vi "T_At_Wire_Err.vi"(8 "InitClock(ms)":u32, 11 "error in (no error)":errorcluster caption="entrée d'erreur") -> (0 "Clock(ms)":u32, 3 "error out":errorcluster caption="sortie d'erreur", 4 "Delta(ms)":u32)   [LabVIEW 2019]
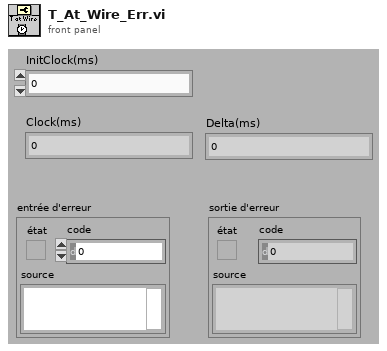
[diagram p1: front panel]
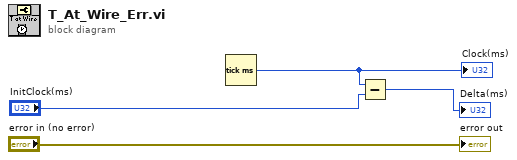
[diagram p0: block diagram]
diagram:
  n1 = Tick Count (ms)() -> (millisecond timer value=w2:u32)
  "Clock(ms)" <- w2
  n2 = Subtract(x=w2, y="InitClock(ms)") -> (x-y=→"Delta(ms)":u32)
  "error out" <- "error in (no error)"
